vi "Read Msg Output.vi"(10 "Msg Output":refnum<class "Msg Output.lvclass">) -> ()   [LabVIEW 2020, in "jettl.lvlib" / "Start jettl Msg.lvlib" / "Start Msg Output.lvlib"]
doc: "jettl 6.14.1.98\nNathan Davis - Nathan Davis\nCopyright (c) 2026, Nathan Davis\nMIT"
uses:
  Start Msg Output.lvlib
  Msg Output/Msg Output.lvclass
  Start Msg Output/Start Msg Output.lvclass
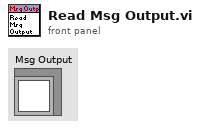
[diagram p1: front panel]
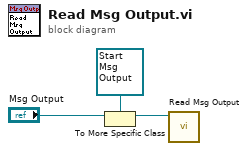
[diagram p0: block diagram]
diagram:
  n1 = To More Specific Class(target class=refnum<class "Start Msg Output.lvclass"> refnum ("_Template.lvlib:Templates.lvlib:TEMPLATE Msg.lvlib:TEMPLATE Msg Output.lvclass"), reference="Msg Output") -> (specific class reference=w1:refnum<class "Start Msg Output.lvclass">)  [unwired: 1 in, 1 out]
  n2 = call "Read Msg Output.vi"("Start Msg Output in"=w1) -> ()  [unwired: 11 in]
